vi "AcquireHardware.vi"(8 "error in (no error)":errorcluster, 11 "ThorLabsCsCamera in":refnum<class "ThorLabsCsCamera.lvclass">) -> (0 "error out":errorcluster, 2 "Image Out":T1, 3 "ThorLabsCsCamera out":refnum<class "ThorLabsCsCamera.lvclass">)   [LabVIEW 2020, in "ThorLabsCsCamera.lvclass"]
uses:
  ThorLabsCsCamera/ThorLabsCsCamera.lvclass
  <vilib>/vision/Image Controls.llb/IMAQ Image.ctl
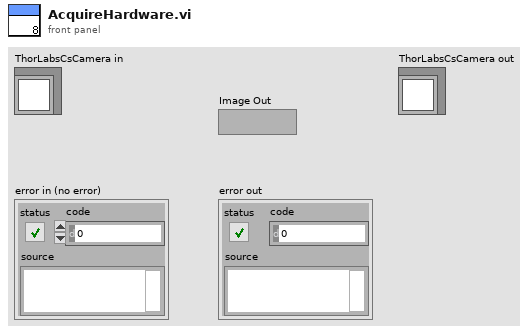
[diagram p1: front panel]
types:
  T1 = typedef "IMAQ Image.ctl" = refnum<image>
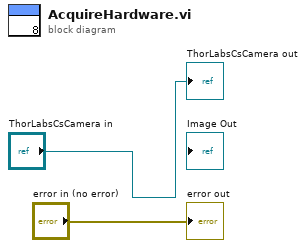
[diagram p0: block diagram]
diagram:
  "error out" <- "error in (no error)"
  "ThorLabsCsCamera out" <- "ThorLabsCsCamera in"
